vi "software_binning.vi"(2 "Input Array":dbl[][](array[numeric])=[[1.0, 2.0, 3.0, 4.0, 5.0, 6.0, 1.0, 2.0], [7.0, 8.0, 9.0, 10.0, 11.0, 12.0, 4.0, 2.0], [13.0, 14.0, 15.0, 16.0, 17.0, 18.0, 60.0, 2.0], [19.0, 20.0, 21.0, 22.0, 23.0, 2.0, 10.0, 2.0], [25.0, 26.0, 27.0, 8.0, 29.0, 3.0, 6.0, 2.0], [31.0, 2.0, 33.0, 4.0, 35.0, 36.0, 5.0, 3.0], [4.0, 8.0, 0.0, 0.0, 0.0, 0.0, 7.0, 3.0], [5.0, 0.0, 0.0, 4.0, 5.0, 0.0, 2.0, 3.0], [50.0, 5.0, 0.0, 0.0, 20.0, 8.0, 5.0, 3.0], [3.0, 2.0, 400.0, 5.0, 10.0, 0.0, 4.0, 11.0], [8.0, 4.0, 5.0, 5.0, 7.0, 1.0, 1.0, 11.0], [4.0, 3.0, 1.0, 4.0, 42.0, 20.0, 8.0, 23.0]], 3 "bin size":u16=1) -> (0 "Binned Array":dbl[][](array[numeric]))   [LabVIEW 2016]
panel:
  out "SubArray - \npoints binned together":i32[][](array[numeric])
  out "Size of Input Array":i32[](array[numeric])
  out "Binned Image":dbl[][](graph)
  out "Uncut Image":dbl[][](graph)
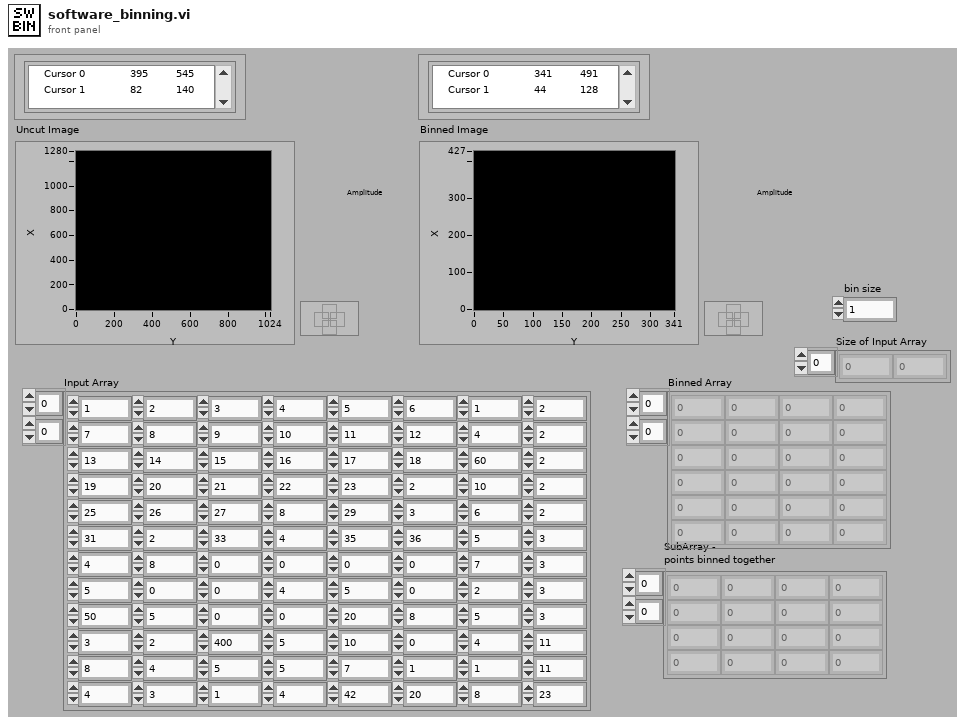
[diagram p1: front panel]
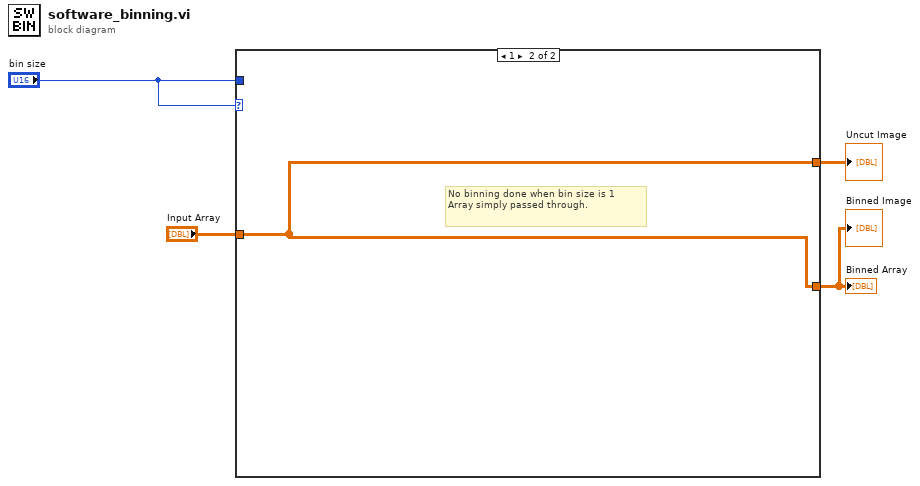
[diagram p0: block diagram]
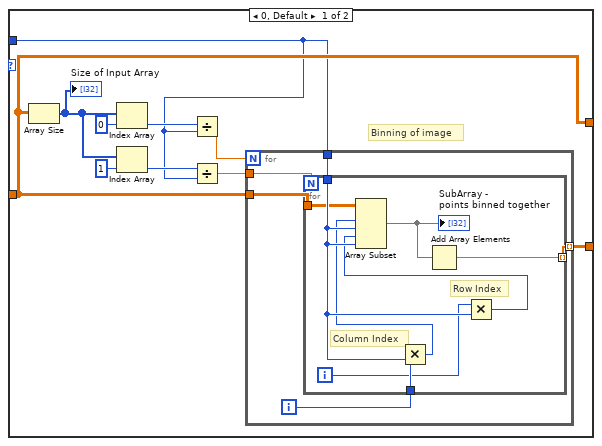
[diagram p2: hidden frame]
diagram:
  n1 = case shown="1" "bin size" {
    tunnel: [w7 w28] -> w4
    tunnel: "Input Array" -> [w6 w28]
    tunnel: [w6 w28] -> w2
    tunnel: "bin size" -> [w5 _]
    frame 0, Default {
      # "Binning of image"
      n2 = Array Size(array=w6) -> (size(s)=w12:i32[])
      "Size of Input Array" <- w12
      n3 = Index Array(array=w12, index=0) -> (element=w10:i32)
      n4 = Index Array(array=w12, index=1) -> (element=w9:i32)
      n5 = Divide(x=w10, y=w5) -> (x/y=w11:dbl)
      n6 = Divide(x=w9, y=w5) -> (x/y=w8:dbl)
      n7 = for {
        N: w11 -> [_]
        tunnel: w6 -> [w18]
        tunnel: w8 -> [w19]
        tunnel: w5 -> [w17]
        tunnel: [w16] -> w7 mode=indexing
        i -> [w15]
        n8 = for {
          N: w19 -> [_]
          tunnel: w18 -> [w26]
          tunnel: w17 -> [w27]
          tunnel: w15 -> [w25]
          tunnel: [w24] -> w16 mode=indexing
          i -> [w23]
          # "Row Index"
          # "Column Index"
          n9 = Multiply(x=w25, y=w27) -> (x*y=w21:i32)
          n10 = Multiply(x=w23, y=w27) -> (x*y=w20:i32)
          n11 = Array Subset(array=w26, index (row)=w21, length (row)=w27, index (col)=w20, length (col)=w27) -> (w22:dbl[][])
          "SubArray - \npoints binned together" <- w22
          n12 = Add Array Elements(numeric array=w22) -> (sum=w24:dbl)
        }
      }
    }
    frame 1 {
      # "No binning done when bin size is 1\nArray simply passed through."
    }
  }
  "Binned Image" <- w4
  "Uncut Image" <- w2
  "Binned Array" <- w4
